vi "RT_Force mode_Oct24.vi"() -> ()   [LabVIEW 2018]
uses:
  RT/meas mass.ctl
  <vilib>/Analysis/baseanly.llb/Mean (DBL).vi
  <vilib>/FPGAPlugInAG/myRIO-1900/niLvFpga_Open_myRIO-1900.vi
  <vilib>/rvi/interface/common/dynamic/niFpgaDynamicAddResources.vi
  <vilib>/Utility/error.llb/Error Cluster From Error Code.vi
  <vilib>/rvi/errors/niLvFpgaAdjustHostInterfaceError.vi
  <vilib>/addons/control/pid/pid.llb/PID (DBL).vi
  <vilib>/FPGAPlugInAG/Dynamic/niLvFpga_Close_Dynamic.vi
  <vilib>/rvi/interface/nirviOpenFPGA/nirviOpenFPGA.xnode
  UNCC Watt balance Oct19/FPGA Bitfiles/UNCCWattbalanceO_FPGATarget_fpganestedFORW&R_aHmrZ4eE-L4.lvbitx
  FPGA files/fpga_nestedFOR_W&R_ADC_W_2DACs_Write_then_CLK.vi
  <vilib>/rvi/interface/nirviReadWriteControl/nirviReadWriteControl.xnode
  <vilib>/rvi/interface/nirviCloseFPGA/nirviCloseFPGA.xnode
  NiFpgaLv.dll
  <vilib>/rvi/interface/Simulation/niFpgaSimulationCallBeginRW.vi
  <vilib>/addons/control/pid/NI_PID_pid.lvlib
  <vilib>/Analysis/NI_AALBase.lvlib
panel:
  in  "setpoint(um)":dbl format="%.2f"
  in  "PID gains":cluster{"Kp":dbl, "Ki":dbl, "Kd":dbl}={"Kp"=0.0002, "Ki"=0.0001, "Kd"=0.0}
  out "n meas":i32
  out "n tare":i32
  in  "BL (V/m/s)":dbl format="%.2f"
  in  "n moving avg":i32=5
  in  "STOP":bool
  in  "calculate":bool
  in  "reset":bool
  in  "take tare":bool
  in  "take mass":bool
  out "average mass (g)":dbl=308.4781817952617 format="%.3g"
  out "current mass (g)":dbl=308.4781817952617 format="%.3g"
  out "PID Error":dbl(graph) caption="Waveform Chart - Dark"
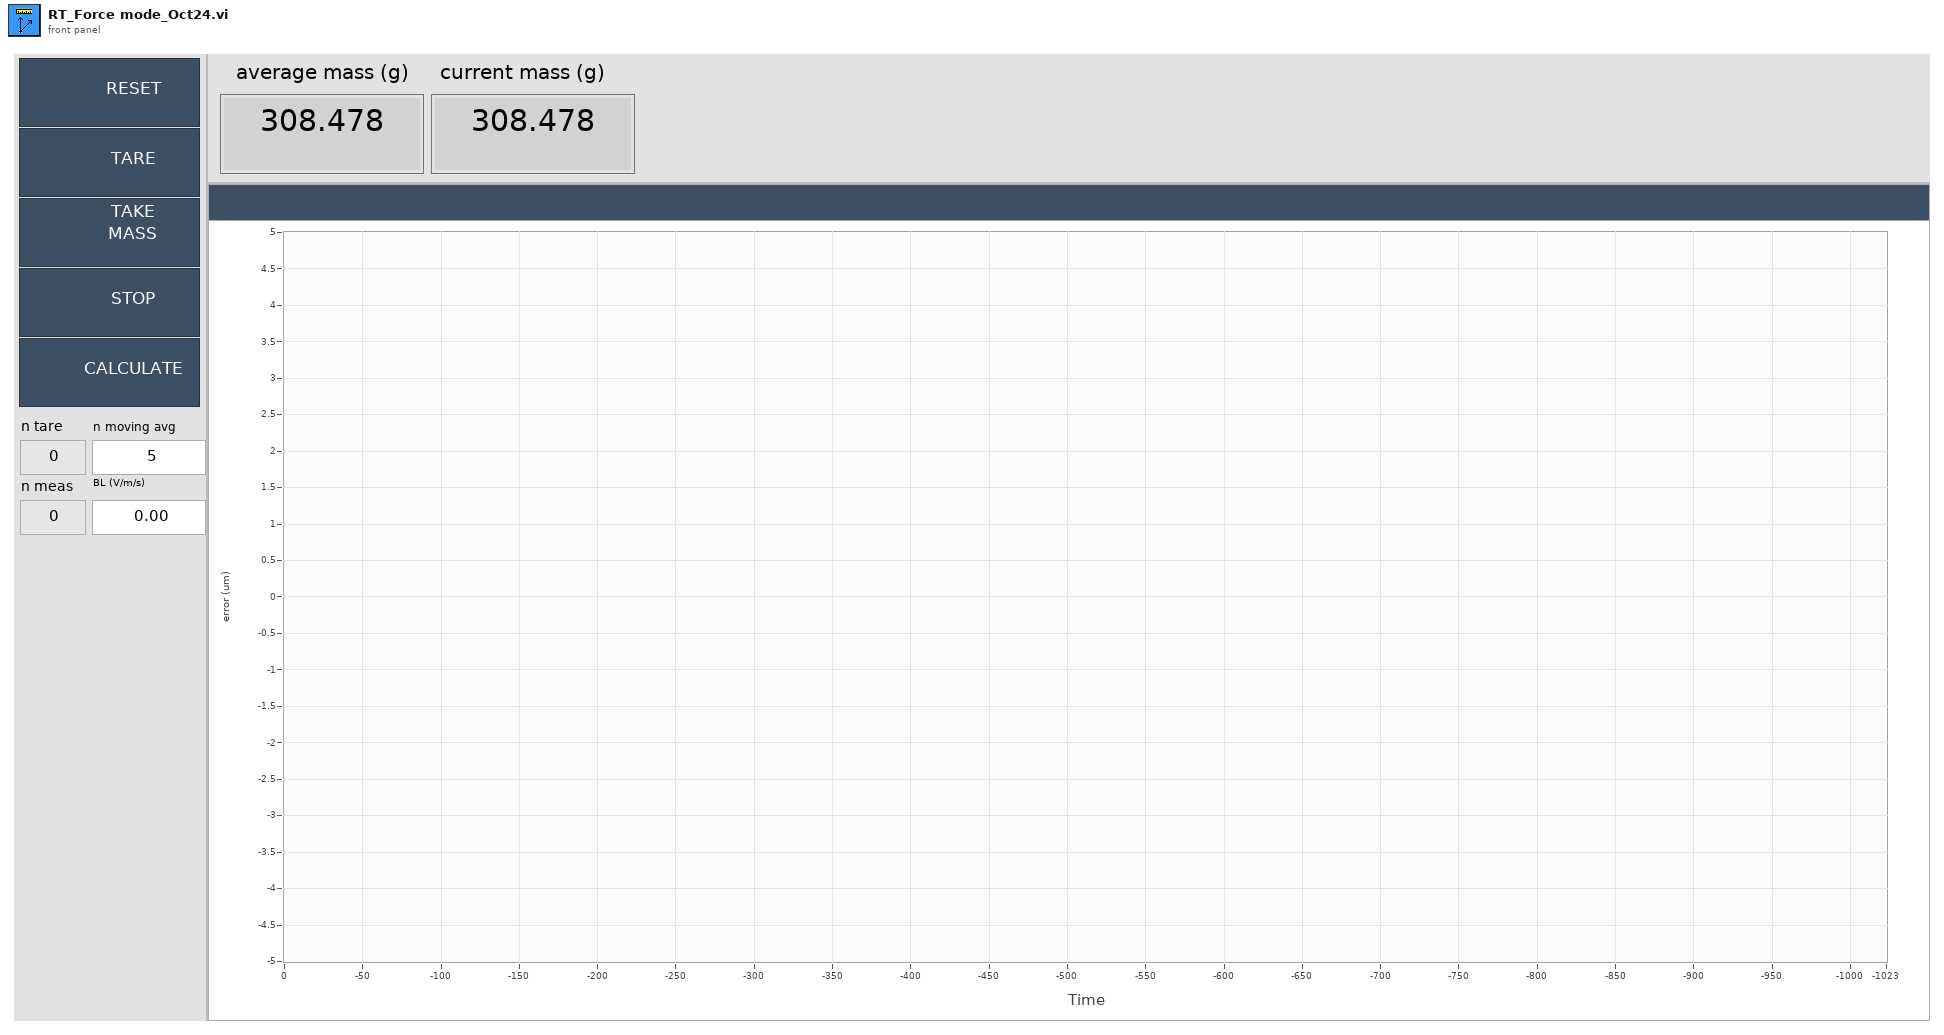
[diagram p1: front panel]
types:
  T1 = typedef "meas mass.ctl" = enum16{"idle", "tare", "take mass", "calculate", "reset"}
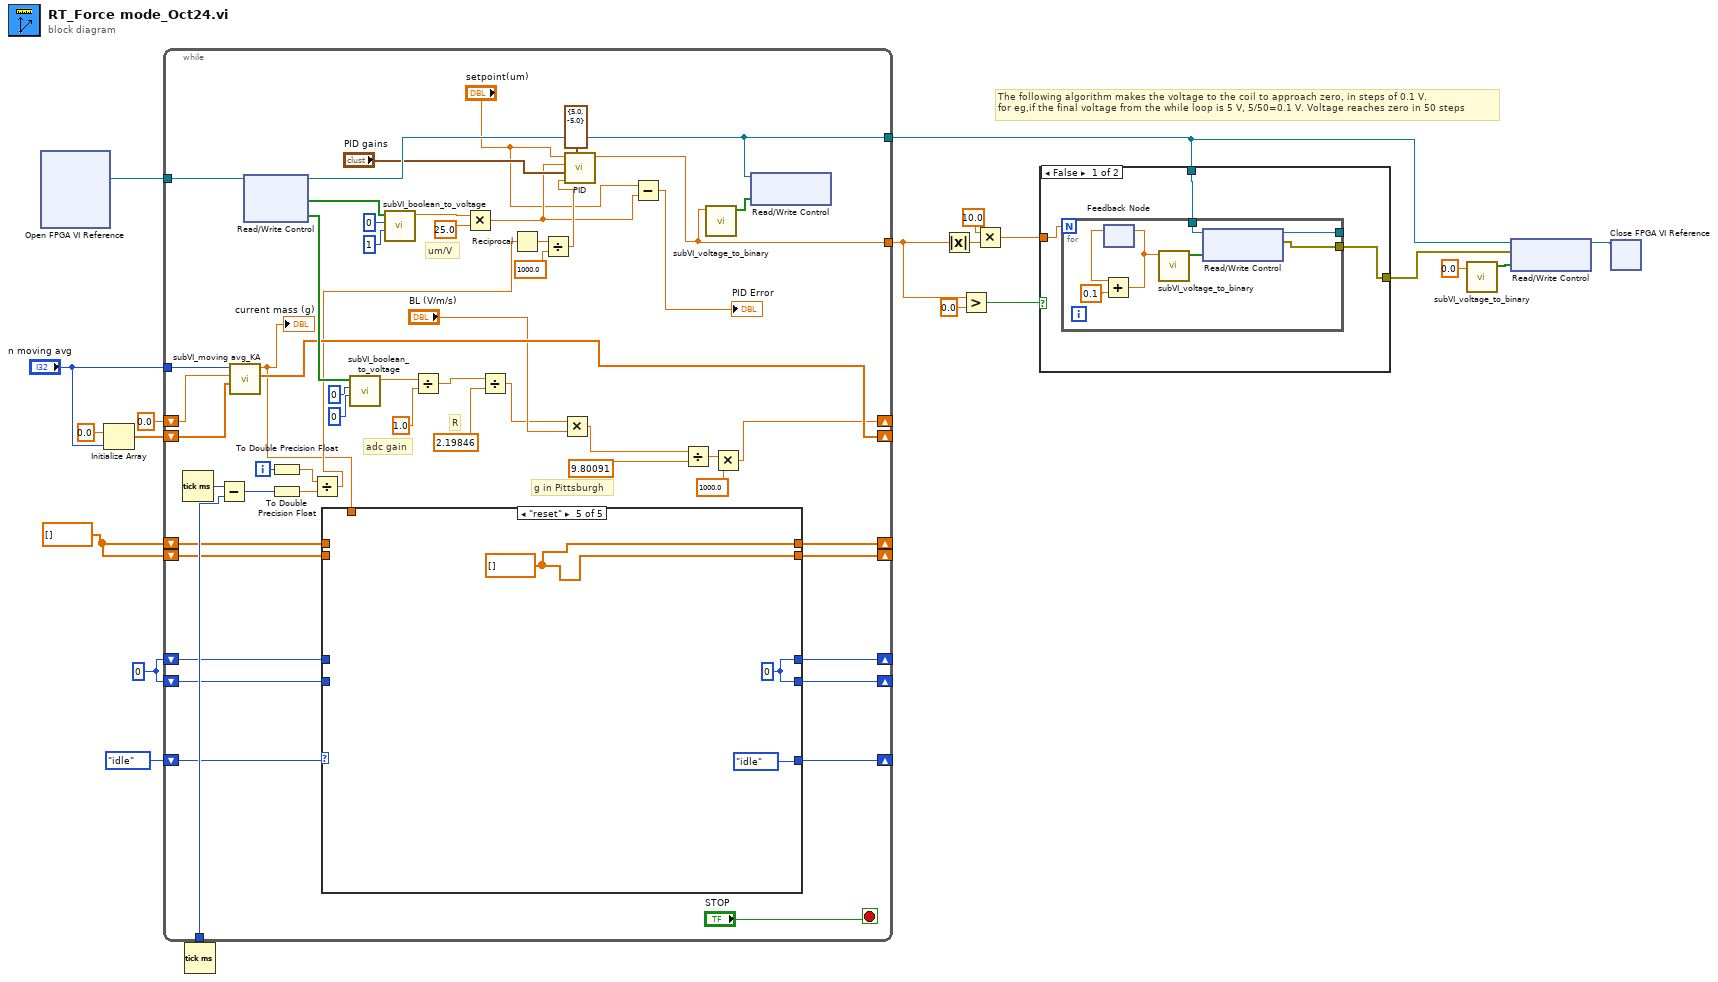
[diagram p0: block diagram]
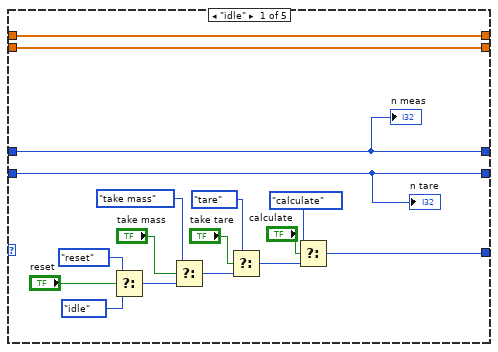
[diagram p2: hidden frame]
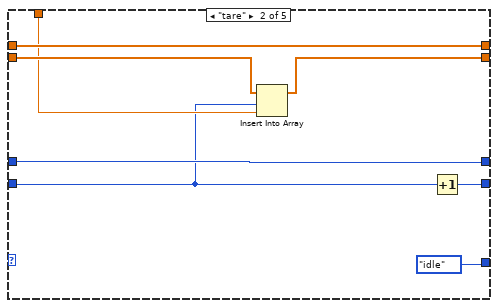
[diagram p3: hidden frame]
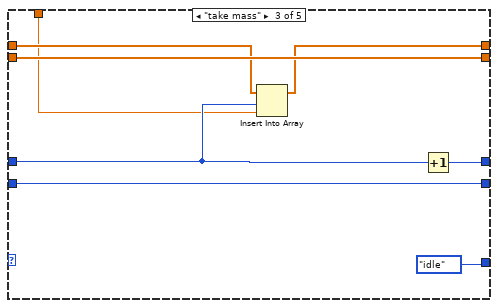
[diagram p4: hidden frame]
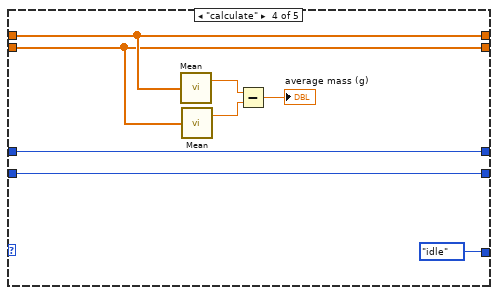
[diagram p5: hidden frame]
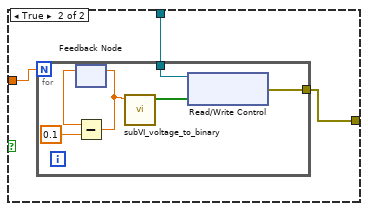
[diagram p6: hidden frame]
diagram:
  w1 = dbl[] []
  w2 = 0
  # "The following algorithm makes the voltage to the coil to approach zero, in steps of 0.1 V.\nfor eg,if the final voltage from the while loop is 5 V, 5/50=0.1 V. Voltage reaches zero in 50 steps"
  n1 = xnode "Open FPGA VI Reference"() -> ("FPGA VI Reference Out"=w14:refnum<k20>)  [unwired: 2 in, 1 out]
  n2 = Initialize Array(0.0 ("element"), "n moving avg") -> (w6:dbl[])
  n3 = Tick Count (ms)() -> (millisecond timer value=w15:u32)
  n4 = while {
    tunnel: w14 -> [w74]
    tunnel: w15 -> [w69]
    tunnel: [w48] -> w13
    tunnel: [w24] -> w8
    tunnel: "n moving avg" -> [w52]
    shift-right: [w41] -> _
    shift-left: 0.0 ("initiation") -> [w51]
    shift-right: [w49] -> _
    shift-left: w6 -> [w50]
    shift-right: [w36] -> _
    shift-left: w1 -> [w37]
    shift-right: [w34] -> _
    shift-left: w1 -> [w33]
    shift-right: [w31] -> _
    shift-left: w2 -> [w32]
    shift-right: [w29] -> _
    shift-left: w2 -> [w30]
    shift-right: [w28] -> _
    shift-left: meas_mass."idle" ("meas mass") -> [w35]
    i -> [w68]
    stop <- "STOP" stop-if-true
    # "adc gain"
    # "R"
    # "g in Pittsburgh"
    # "um/V"
    n5 = Tick Count (ms)() -> (millisecond timer value=w70:u32)
    n6 = Subtract(x=w70, y=w69) -> (x-y=w73:u32)
    n7 = call "subVI_moving avg_KA.vi"("input array"=w50, "sample"=w51, "no. moving avg."=w52) -> ("output array"=w49:dbl[], "avg."=w26:dbl)  [unwired: 7 in]
    "current mass (g)" <- w26
    n8 = xnode "Read/Write Control"("FPGA VI Reference In"=w74) -> ("FPGA VI Reference Out"=w48:refnum<k20>, "ADC  1 R"=w67:bool[], "ADC 4 R"=w66:bool[])  [unwired: 1 in, 1 out]
    n9 = To Double Precision Float(number=w68) -> (double precision float=w72:dbl)
    n10 = To Double Precision Float(number=w73) -> (double precision float=w71:dbl)
    n11 = Divide(x=w72, y=w71) -> (x/y=w40:dbl)
    n12 = case shown="\"reset\"" w35 {
      tunnel: w37 -> [w78 w98 w101 w112 _]
      tunnel: [w78 w98 w102 w112 w116] -> w36
      tunnel: [w77 w96 w107 w111 w116] -> w34
      tunnel: w33 -> [w77 w97 w107 w111 _]
      tunnel: w32 -> [w75 w93 w104 w115 _]
      tunnel: [w75 w93 w105 w115 w117] -> w31
      tunnel: w30 -> [w76 w92 w103 w114 _]
      tunnel: [w76 w94 w103 w114 w117] -> w29
      tunnel: [w79 meas_mass."idle" ("meas mass") meas_mass."idle" ("meas mass") meas_mass."idle" ("meas mass") meas_mass."idle" ("meas mass")] -> w28
      tunnel: w26 -> [_ w95 w100 _ _]
      frame "idle" {
        n13 = Select(t=meas_mass."reset" ("meas mass"), s="reset", f=meas_mass."idle" ("meas mass")) -> (s? t:f=w88:T1)
        n14 = Select(t=meas_mass."take mass" ("meas mass"), s="take mass", f=w88) -> (s? t:f=w85:T1)
        n15 = Select(t=meas_mass."tare" ("meas mass"), s="take tare", f=w85) -> (s? t:f=w81:T1)
        n16 = Select(t=meas_mass."calculate" ("meas mass"), s="calculate", f=w81) -> (s? t:f=w79:T1)
        "n tare" <- w76
        "n meas" <- w75
      }
      frame "tare" {
        n17 = Insert Into Array(array=w97, index=w92, new element=w95) -> (w96:dbl[])
        n18 = Increment(x=w92) -> (x+1=w94:i32)
      }
      frame "take mass" {
        n19 = Insert Into Array(array=w101, index=w104, new element=w100) -> (w102:dbl[])
        n20 = Increment(x=w104) -> (x+1=w105:i32)
      }
      frame "calculate" {
        n21 = call-poly <vilib>:"Mean.vi"("X"=w112) -> ("mean"=w110:dbl)  [unwired: 1 out]
        n22 = call-poly <vilib>:"Mean.vi"("X"=w111) -> ("mean"=w109:dbl)  [unwired: 1 out]
        n23 = Subtract(x=w110, y=w109) -> (x-y=→"average mass (g)":dbl)
      }
      frame "reset" {
        w116 = dbl[] []
        w117 = 0
      }
    }
    n24 = call "subVI_boolean_to_voltage.vi"("Gain"=i16 0, "UNI"=i16 0, "ADC read"=w66) -> ("V"=w57:dbl)  [unwired: 8 in]
    n25 = call "subVI_boolean_to_voltage.vi"("Gain"=i16 1, "UNI"=i16 0, "ADC read"=w67) -> ("V"=w62:dbl)  [unwired: 8 in]
    n26 = Divide(x=w57, y=1.0 ("ADC gain")) -> (x/y=w46:dbl)
    n27 = Multiply(x=w62, y=25.0) -> (x*y=w22:dbl)
    n28 = Divide(x=w46, y=2.19846 ("R")) -> (x/y=w38:dbl)
    n29 = Reciprocal(x=w40) -> (1/x=w43:dbl)
    n30 = Divide(x=w43, y=1000.0) -> (x/y=w25:dbl)
    n31 = Multiply(x=w38, y="BL (V/m/s)") -> (x*y=w56:dbl)
    n32 = call-poly <vilib>:"PID.vi"("output range"=cluster{"output high":dbl, "output low":dbl} {"output high"=5.0, "output low"=-5.0}, "dt (s)"=w25, "PID gains"="PID gains", "process variable"=w22, "setpoint"="setpoint(um)") -> ("output"=w24:dbl)  [unwired: 5 in, 1 out]
    n33 = Subtract(x="setpoint(um)", y=w22) -> (x-y=→"PID Error":dbl)
    n34 = Divide(x=w56, y=9.80091) -> (x/y=w54:dbl)
    n35 = call "subVI_voltage_to_binary.vi"("voltage"=w24) -> ("binary"=w47:bool[])  [unwired: 10 in]
    n36 = Multiply(x=w54, y=1000.0) -> (x*y=w41:dbl)
    n37 = xnode "Read/Write Control"("FPGA VI Reference In"=w48, "DAC 1 write"=w47) -> ()  [unwired: 1 in, 2 out]
  }
  n38 = Absolute Value(x=w8) -> (abs(x)=w16:dbl)
  n39 = Greater?(x=w8, y=0.0) -> (0:w20:bool)
  n40 = Multiply(x=10.0, y=w16) -> (x*y=w19:dbl)
  n41 = case shown="False" w20 {
    tunnel: w19 -> [w121 w131]
    tunnel: w13 -> [w120 w130]
    tunnel: [w119 w129] -> w9
    frame False {
      n42 = for {
        N: w121 -> [_]
        tunnel: [w127] -> _
        tunnel: [w123] -> w119
        tunnel: w120 -> [w122]
        n43 = feedback #1() -> (w125:dbl)  [unwired: 1 in]
        n44 = Add(x=w125, y=0.1) -> (x+y=w124:dbl)
        n45 = feedback-in #1(w124) -> ()
        n46 = call "subVI_voltage_to_binary.vi"("voltage"=w124) -> ("binary"=w128:bool[])  [unwired: 10 in]
        n47 = xnode "Read/Write Control"("FPGA VI Reference In"=w122, "DAC 1 write"=w128) -> ("FPGA VI Reference Out"=w127:refnum<k20>, "error out"=w123:errorcluster)  [unwired: 1 in]
      }
    }
    frame True {
      n48 = for {
        N: w131 -> [_]
        tunnel: [w133] -> w129
        tunnel: w130 -> [w132]
        n49 = feedback #2() -> (w136:dbl)  [unwired: 1 in]
        n50 = Subtract(x=w136, y=0.1) -> (x-y=w134:dbl)
        n51 = feedback-in #2(w134) -> ()
        n52 = call "subVI_voltage_to_binary.vi"("voltage"=w134) -> ("binary"=w137:bool[])  [unwired: 10 in]
        n53 = xnode "Read/Write Control"("FPGA VI Reference In"=w132, "DAC 1 write"=w137) -> ("error out"=w133:errorcluster)  [unwired: 1 in, 1 out]
      }
    }
  }
  n54 = call "subVI_voltage_to_binary.vi"("voltage"=0.0) -> ("binary"=w11:bool[])  [unwired: 10 in]
  n55 = xnode "Read/Write Control"("FPGA VI Reference In"=w13, "error in"=w9, "DAC 1 write"=w11) -> ("FPGA VI Reference Out"=w12:refnum<k20>)  [unwired: 1 out]
  n56 = xnode "Close FPGA VI Reference"("FPGA VI Reference In"=w12) -> ()  [unwired: 1 in, 1 out]
